vi "SoftwareGate_Rapid Read.vi"(0 "Timeout (s)":dbl, 1 "Channel":string="1", 2 "Digitizer Settings":T5={"Digitizer delay (us) "=0.0, "rf points per line"=2048, "lines per plane"=128, "Samp Rate (Hz)"=100000000.0, "Additional dig delay (us)"=0.0, "Voltage Scale"=0.4, "Pre-Looks"=0, "Offset delay (us)"=0.0, "bits A/D"=8, "Avg Num"=1, "DigTimeOut"=5.0, "Rel Dig Delay"=0.0, "Dig Ch"=0, "LeCroyCluster"={"LeCroy Channels"=[TRUE, FALSE, FALSE, FALSE], "LC read pt offset"=0.0, "Sweep Avg"=FALSE}, "Main Digitizer"=enum."NI Digitizer", "Dig Config"=enum."Single channel", "Digitizer ID Cluster"={"Acqiris/Alazar/SP ID"=[], "NI Instr Handles"=[], "LeCroy VISA"="", "GaGe Handle"={"Handle"=0, "Sample size"=0, "Resolution"=0, "Offset"=0, "Channels"=0, "Boards"=0}, "ATS Ref"="ATS9350", "Acqiris Address"=["PCI::INSTR0"], "ADQRef"=refnum, "adq_cu_ptr"=refnum}, "Trigger Settings"={"Trig Source"=1, "Trig Coupling"=0, "Trig Slope"=0, "Level (mV)"=1500.0}, "Bulk Acq"=FALSE, "Bulk Start Indexes"=[], "Data Ref RF"=refnum, "NI ID/Channel"=[], "Total Dig CH"=5, "Xtra Ann Trig delay (us)"=10.0, "Fix Z Delay?"=FALSE, "One Way Transmission?"=FALSE, "Data Ref Log"=refnum} {"Trigger Settings"."Trig Slope" items=["Positive", "Negative"]; "Trigger Settings"."Level (mV)" format="%.2f"; "Trigger Settings"."Trig Coupling" items=["DC 1 MOhm", "AC 1 MOhm", "DC 50 Ohm", "AC 50 Ohm"]; "Trigger Settings"."Trig Source" items=["Chan 1", "External"]; "Rel Dig Delay" format="%.2f"; "DigTimeOut" format="%.2f"; "Avg Num" min=1; "Offset delay (us)" format="%.2f"; "Additional dig delay (us)" format="%.2f"; "Digitizer delay (us)" format="%.2f"}, 7 "AlazarCluster":T9, 9 "Motion Settings":T1={"No Motion?"=FALSE, "Motion System"=enum."NI 735x", "Motion Bd ID"=1, "Motion Profile"="SMAC1", "# Axis"=1, "Reverse Z axis?"=TRUE, "SMAC Axis"=0, "scan pair"=enum."y-(x) scan", "RT fps"=6.0, "Steps per mm"=[1000, 1000, 1000, 1000], "Motor Parameters"={"velocity ct/s"=[10000.0, 10000.0, 10000.0, 50000.0], "accel ct/s^2"=[50000.0, 50000.0, 50000.0, 200000.0]}, "One Way Scan"=FALSE, "Reverse One Way Scan"=FALSE, "Global Position (mm)"=[], "Plane"=0, "Distance between\nscan lines (um)"=0.0, "Distance between\nscan planes (um)"=0.0, "number of scan planes"=1, "Total steps in line"=0, "Xtra plane\ndistance  (um)"=100, "Xtra planes "=1, "Add Axis"=FALSE, "overshoot cts"=200, "BKPT Shift"=0, "Scan Start Time (ms)"=0, "ESP VISA"="GPIB::1::INSTR", "3rd Axis"=1, "GL Ref Out"=refnum, "Galil Address"=""} {"3rd Axis" items=["x", "y", "z", "w"]; "Xtra planes" min=1; "Xtra plane\ndistance  (um)" min=0; "Distance between\nscan planes (um)" format="%.2f"; "Distance between\nscan lines (um)" format="%.2f"; "SMAC Axis" items=["None"=0, "Axis 1"=1, "Axis 2"=2, "Axis 3"=3, "Axis 4"=4, "Axis 5"=5, "Axis 6"=6, "Axis 7"=7, "Axis 8"=8, "Vector Space 1"=17, "Vector Space 2"=18, "Vector Space 3"=19, "Vector Space 4"=20]; "Motion Bd ID" min=1 max=32 step=1}, 11 "error in":errorcluster, 14 "Software Gate":bool) -> (3 "gain":dbl, 4 "Array":i16[][](array[numeric]), 6 "Reverse?":bool, 15 "error out":errorcluster)   [LabVIEW 2022 SP3]
uses:
  ScanningControl/Digitizers/-DigitizerRoutines/DigitizerSettings.ctl
  ScanningControl/Digitizers/-DigitizerRoutines/Digitizer.ctl
  ScanningControl/Digitizers/-DigitizerRoutines/DigConfig.ctl
  ScanningControl/Digitizers/-DigitizerRoutines/DigitizerID.ctl
  C:/Windows/System32/ADQAPI_dotNet_helper.dll
  ScanningControl/Motion Controllers/NI_controller/-NI_MotionRoutines/MotionParameters.ctl
  ScanningControl/Motion Controllers/NI_controller/-NI_MotionRoutines/MotionSys.ctl
  ScanningControl/Motion Controllers/-MotionRoutines/ScanAxis.ctl
  ScanningControl/Motion Controllers/-MotionRoutines/3rdAxis.ctl
  <vilib>/DAQmx/write.llb/DAQmx Write (Digital Bool 1Line 1Point).vi
  ScanningControl/Motion Controllers/-MotionRoutines/MotionGlobals.vi
  <vilib>/DAQmx/miscellaneous.llb/DAQmx Fill In Error Info.vi
  <instrlib>/niScope/Acquire/Fetch/niScope Multi Fetch Binary 8.vi
  <instrlib>/Acqiris Dx/Acqiris Dx.lvlib
panel:
  # "1-D and 2-D B scan settings"
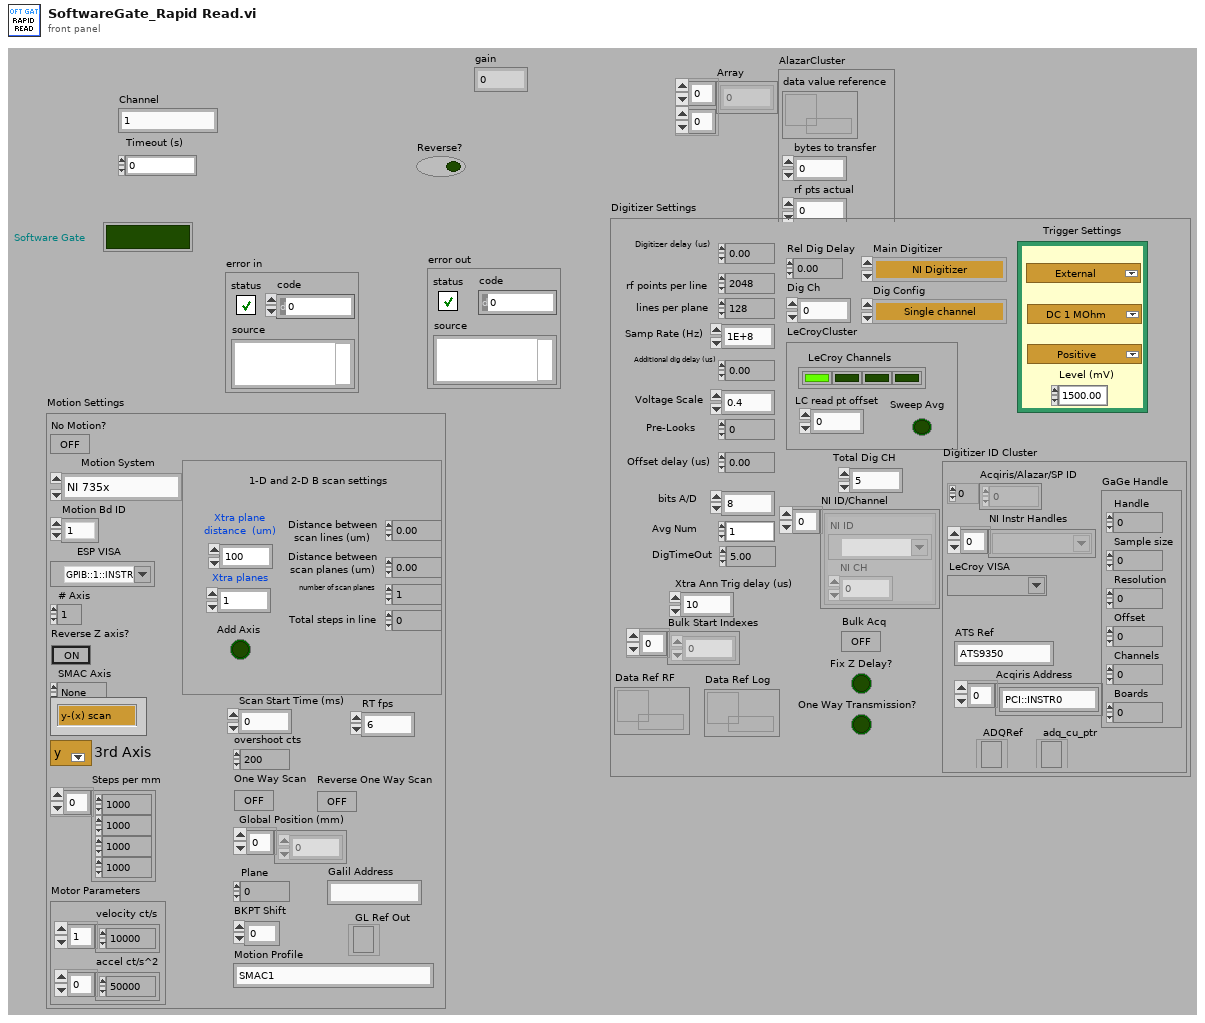
[diagram p1: front panel]
types:
  T1 = typedef "MotionParameters.ctl" = cluster{"No Motion?":bool, "Motion System":T2, "Motion Bd ID":u8, "Motion Profile":string, "# Axis":i8, "Reverse Z axis?":bool, "SMAC Axis":u16, "scan pair":T3, "RT fps":sgl, "Steps per mm":i32[], "Motor Parameters":cluster{"velocity ct/s":dbl[], "accel ct/s^2":dbl[]}, "One Way Scan":bool, "Reverse One Way Scan":bool, "Global Position (mm)":dbl[], "Plane":i32, "Distance between\nscan lines (um)":sgl, "Distance between\nscan planes (um)":sgl, "number of scan planes":i32, "Total steps in line":i32, "Xtra plane\ndistance  (um)":i32, "Xtra planes ":i32, "Add Axis":bool, "overshoot cts":i32, "BKPT Shift":i32, "Scan Start Time (ms)":u32, "ESP VISA":refnum<visa-resource-name>, "3rd Axis":T4, "GL Ref Out":refnum<k7>, "Galil Address":string}
  T2 = typedef "MotionSys.ctl" = enum16{"MM3000", "NI 735x", "Newport ESP", "No Motion Card", "Galil"}
  T3 = typedef "ScanAxis.ctl" = enum16{"y-(x) scan", "x-(y) scan", "z-(x) scan", "z-(y) scan", "y-(z) scan", "x-(z) scan", "w-(x) scan", "w-(y) scan", "w-(z) scan", "x-(w) scan", "y-(w) scan", "z-(w) scan"}
  T4 = typedef "3rdAxis.ctl" = u16
  T5 = typedef "DigitizerSettings.ctl" = cluster{"Digitizer delay (us) ":dbl, "rf points per line":i32, "lines per plane":i32, "Samp Rate (Hz)":dbl, "Additional dig delay (us)":dbl, "Voltage Scale":dbl, "Pre-Looks":i32, "Offset delay (us)":dbl, "bits A/D":i8, "Avg Num":i32, "DigTimeOut":sgl, "Rel Dig Delay":sgl, "Dig Ch":i32, "LeCroyCluster":cluster{"LeCroy Channels":bool[], "LC read pt offset":dbl, "Sweep Avg":bool}, "Main Digitizer":T6, "Dig Config":T7, "Digitizer ID Cluster":T8, "Trigger Settings":cluster{"Trig Source":u16, "Trig Coupling":u16, "Trig Slope":u16, "Level (mV)":dbl}, "Bulk Acq":bool, "Bulk Start Indexes":i32[], "Data Ref RF":refnum<data-value>, "NI ID/Channel":cluster{"NI ID":refnum<k15>, "NI CH":i32}[], "Total Dig CH":i32, "Xtra Ann Trig delay (us)":dbl, "Fix Z Delay?":bool, "One Way Transmission?":bool, "Data Ref Log":refnum<data-value>}
  T6 = typedef "Digitizer.ctl" = enum16{"Acqiris Digitizer", "NI Digitizer", "LeCroy", "GaGe", "AlazarTech", "No Digitizer", "Teledyne"}
  T7 = typedef "DigConfig.ctl" = enum16{"Single channel", "2 Chans w/ 2 Acqiris", "2 Chans w/ 1 Acqiris", "5-CH Pulser New", "5-CH pulser w/ ann array", "5-pass style ann array", "Empty"}
  T8 = typedef "DigitizerID.ctl" = cluster{"Acqiris/Alazar/SP ID":u32[], "NI Instr Handles":refnum<k15>[], "LeCroy VISA":refnum<visa-resource-name>, "GaGe Handle":cluster{"Handle":u32, "Sample size":u32, "Resolution":i32, "Offset":i32, "Channels":u32, "Boards":u32}, "ATS Ref":string, "Acqiris Address":string[], "ADQRef":refnum<k24>, "adq_cu_ptr":refnum<k24>}
  T9 = cluster{"data value reference":refnum<data-value>, "bytes to transfer":u32, "rf pts actual":u32}
  T10 = typedef "Var" = u8
  T11 = cluster{"horPos":dbl, "timeStampLo":u32, "timeStampHi":u32}[]
  T12 = cluster{"returnedSamplesPerSeg":i32, "indexFirstPoint":i32, "sampTime":dbl, "vGain":dbl, "vOffset":dbl, "returnedSegments":i32, "nbrAvgWforms":i32, "actualTriggersInAcqLo":u32, "actualTriggersInAcqHi":u32, "reserved3":dbl, "actualDataSize":u32, "missingValue":dbl}
  T13 = typedef "Bd Id Out" = u8
  T14 = cluster{"actualSamples":i32, "absoluteInitialX":dbl, "relativeInitialX":dbl, "xIncrement":dbl, "offset":dbl, "gain":dbl, "reserved1":dbl, "reserved2":dbl}[]
  T15 = cluster{"actualSamples":i32, "absoluteInitialX":dbl, "relativeInitialX":dbl, "xIncrement":dbl, "offset":dbl, "gain":dbl, "reserved1":dbl, "reserved2":dbl}
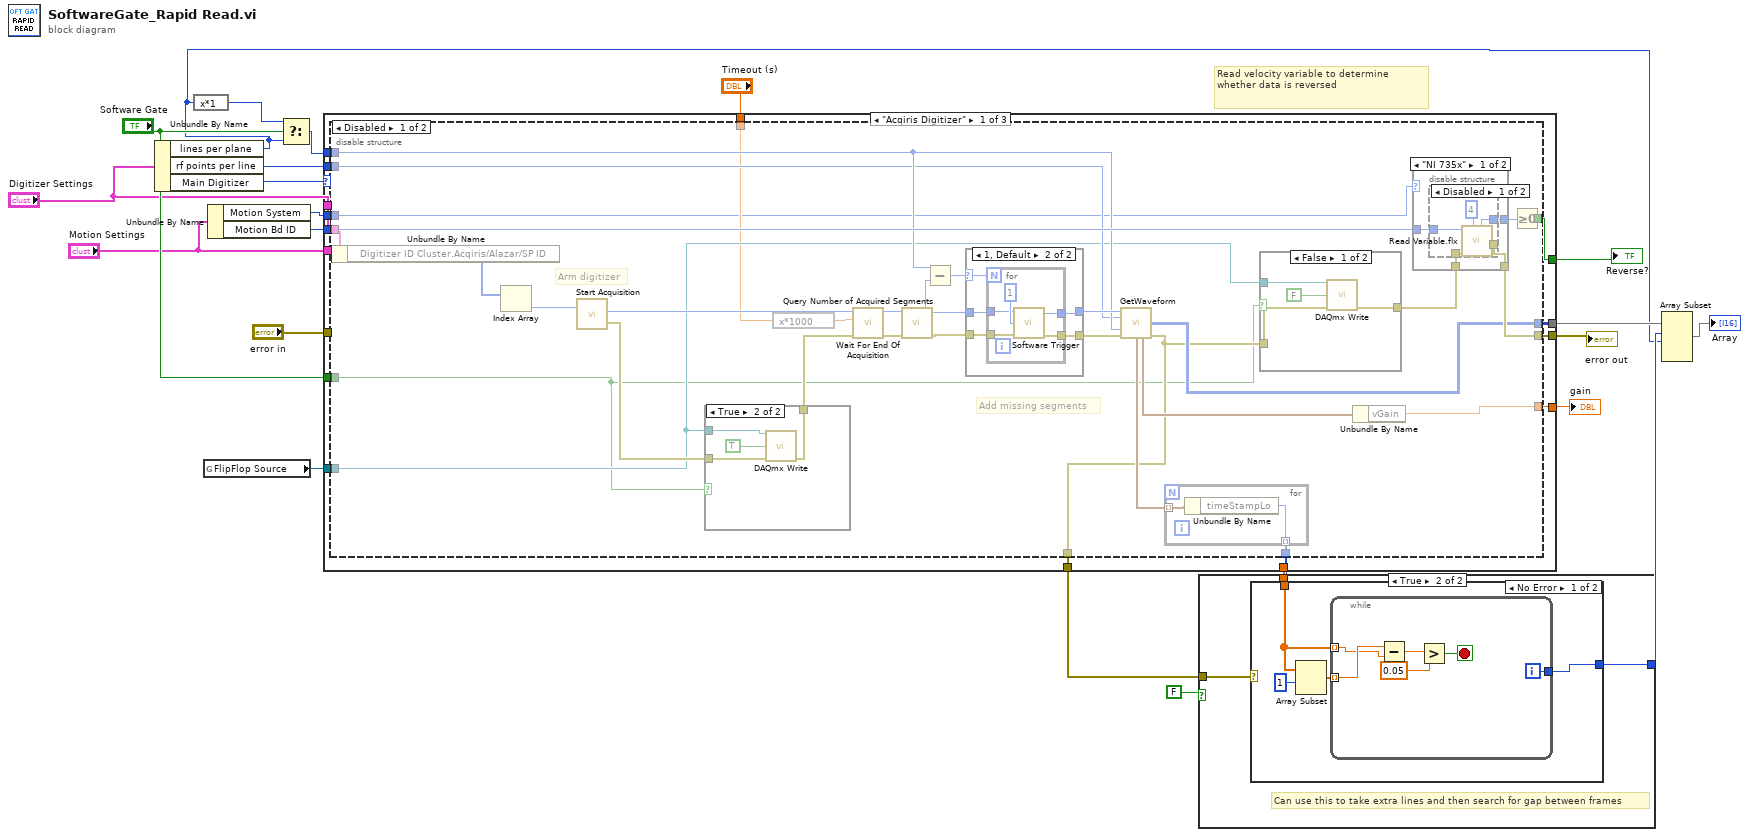
[diagram p0: block diagram]
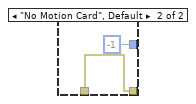
[diagram p7: hidden frame]
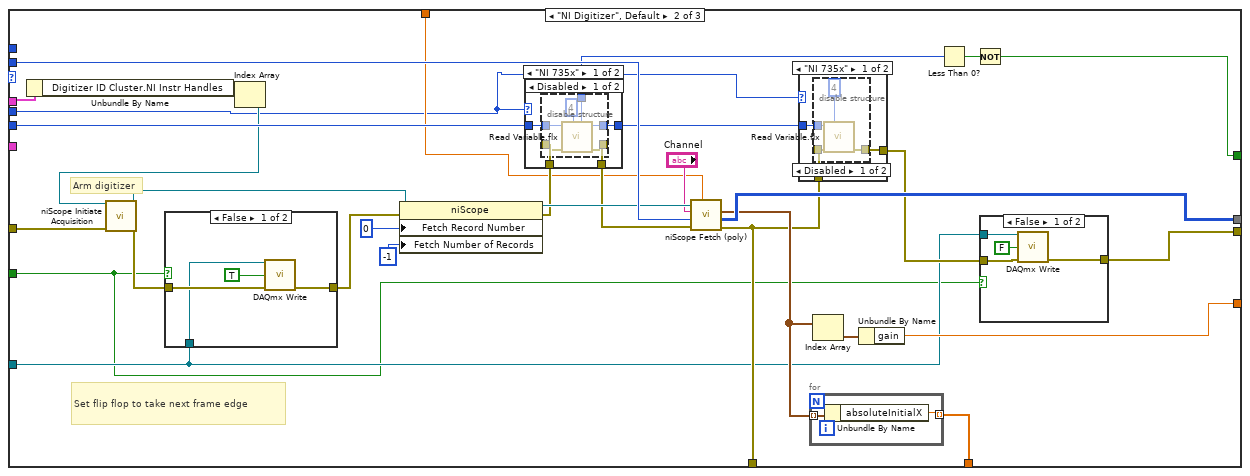
[diagram p10: hidden frame]
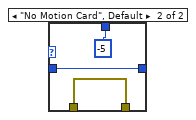
[diagram p16: hidden frame]
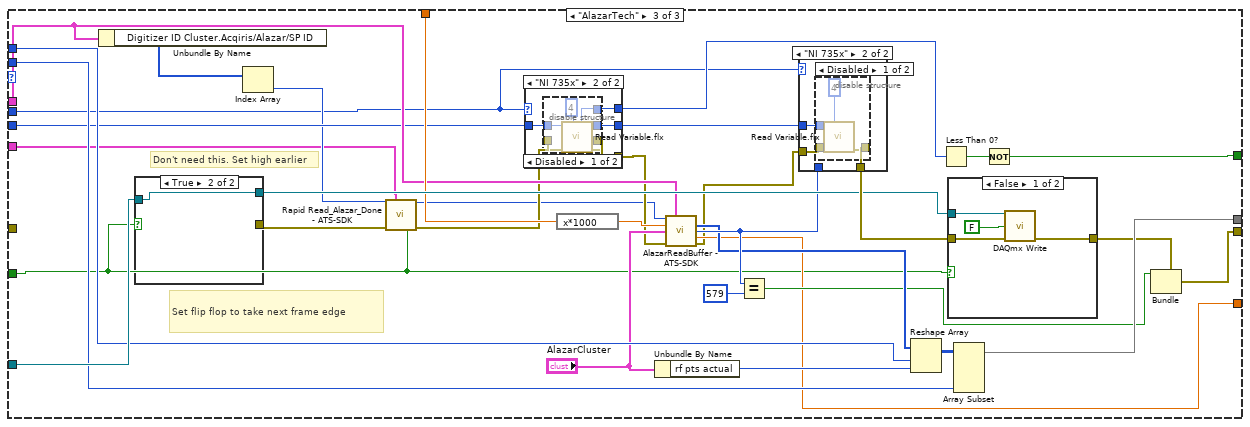
[diagram p17: hidden frame]
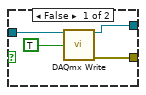
[diagram p18: hidden frame]
diagram:
  # "Read velocity variable to determine whether data is reversed"
  n1 = Unbundle By Name("Digitizer Settings") -> ("lines per plane"=w4:i32, "rf points per line"=w5:i32, "Main Digitizer"=w6:T6)
  n2 = expression code="x*1"(w4) -> (w16:i32)
  n3 = global read "MotionGlobals.vi" "FlipFlop Source"() -> (w18:refnum<k21>)
  n4 = Unbundle By Name("Motion Settings") -> ("Motion System"=w1:T2, "Motion Bd ID"=w2:u8)
  n5 = Select(t=w16, s="Software Gate", f=w4) -> (s? t:f=w15:i32)
  n6 = case shown="\"Acqiris Digitizer\"" w6 {
    tunnel: [w36 w107 w185] -> w22
    tunnel: w2 -> [w34 w133 w173]
    tunnel: "error in" -> [_ w131 _]
    tunnel: w5 -> [w32 w134 w194]
    tunnel: w15 -> [w33 _ w195]
    tunnel: [w31 w119 w193] -> w13
    tunnel: [w35 w116 w197] -> w20
    tunnel: [w30 w125 w182] -> w19
    tunnel: w18 -> [w29 w106 w200]
    tunnel: "Digitizer Settings" -> [w28 w115 w181]
    tunnel: "Timeout (s)" -> [w27 w110 w189]
    tunnel: [w26 w111 _] -> w14
    tunnel: [w25 w109 _] -> w10
    tunnel: "Software Gate" -> [w24 w105 w174]
    tunnel: "Motion Settings" -> [_ _ w170]
    tunnel: w1 -> [w23 w104 w169]
    frame "Acqiris Digitizer" {
      n7 = disable-structure shown="Disabled" {
        disable-tunnel: [w58 _] -> w36
        disable-tunnel: [w57 _] -> w35
        disable-tunnel: w34 -> [w56 _]
        disable-tunnel: w33 -> [w55 _]
        disable-tunnel: w32 -> [w54 _]
        disable-tunnel: [w53 _] -> w31
        disable-tunnel: [w51 _] -> w30
        disable-tunnel: w29 -> [w47 _]
        disable-tunnel: w28 -> [w46 _]
        disable-tunnel: w27 -> [w43 _]
        disable-tunnel: [w41 _] -> w26
        disable-tunnel: [w39 _] -> w25
        disable-tunnel: w24 -> [w38 _]
        disable-tunnel: w23 -> [w37 _]
        frame Disabled {
          # "Arm digitizer"
          # "Add missing segments"
          n8 = Unbundle By Name(w46) -> ("Digitizer ID Cluster.Acqiris/Alazar/SP ID"=w45:u32[])
          n9 = Index Array(array=w45) -> (element=w44:u32)  [unwired: 1 in]
          n10 = call <instrlib>:"Start Acquisition.vi"("Instrument ID"=w44) -> ("error out"=w50:errorcluster, "dup Instrument ID"=w60:u32)  [unwired: 3 in]
          n11 = case shown="True" w38 {
            tunnel: w50 -> [w74 w77]
            tunnel: [w74 w76] -> w49
            tunnel: w47 -> [_ w75]
            frame False {
            }
            frame True {
              n12 = call-poly <vilib>:"DAQmx Write.vi"("task/channels in"=w75, "data"=TRUE ("stop (T)"), "error in"=w77) -> ("error out"=w76:errorcluster)  [unwired: 10 in, 2 out]
            }
          }
          n13 = expression code="x*1000"(w43) -> (w40:dbl)
          n14 = call <instrlib>:"Wait For End Of Acquisition.vi"("error in (no error)"=w49, "Timeout"=w40, "Instrument ID"=w60) -> ("error out"=w61:errorcluster, "dup Instrument ID"=w65:u32)  [unwired: 3 out]
          n15 = call <instrlib>:"Query Number of Acquired Segments.vi"("error in (no error)"=w61, "Instrument ID"=w65) -> ("error out"=w67:errorcluster, "Number of Segments"=w68:i32, "dup Instrument ID"=w64:u32)  [unwired: 3 out]
          n16 = Subtract(x=w55, y=w68) -> (x-y=w63:i32)
          n17 = case shown="1, Default" w63 {
            selector: w63 -> [_ w94]
            tunnel: w67 -> [w92 w98]
            tunnel: [w92 w97] -> w66
            tunnel: w64 -> [w93 w96]
            tunnel: [w93 w95] -> w62
            frame 0 {
            }
            frame 1, Default {
              n18 = for {
                N: w94 -> [_]
                tunnel: w98 -> [w103]
                tunnel: w96 -> [w100]
                tunnel: [w102] -> w97
                tunnel: [w99] -> w95
                n19 = call <instrlib>:"Software Trigger.vi"("error in (no error)"=w103, "Type"=1, "Instrument ID"=w100) -> ("error out"=w102:errorcluster, "dup Instrument ID"=w99:u32)
              }
            }
          }
          n20 = call "GetWaveform.vi"("Acq ID Out"=w62, "Num Samps"=w54, "Num Segs"=w55, "error in"=w66) -> ("Acquired Waveform16 bit"=w53:i16[][], "segDescArray out"=w42:T11, "dataDesc"=w52:T12, "error out"=w39:errorcluster)  [unwired: 2 in, 6 out]
          n21 = for {
            tunnel: w42 -> [w80] mode=indexing
            tunnel: [w79] -> w41 mode=indexing
            n22 = Unbundle By Name(w80) -> ("timeStampLo"=w79:u32)
          }
          n23 = case shown="False" w38 {
            tunnel: [w71 w73] -> w48
            tunnel: w47 -> [w70 _]
            tunnel: w39 -> [w69 w73]
            frame False {
              n24 = call-poly <vilib>:"DAQmx Write.vi"("task/channels in"=w70, "data"=FALSE ("stop (T)"), "error in"=w69) -> ("error out"=w71:errorcluster)  [unwired: 10 in, 2 out]
            }
            frame True {
            }
          }
          n25 = Unbundle By Name(w52) -> ("vGain"=w51:dbl)
          n26 = case shown="\"NI 735x\"" w37 {
            tunnel: [w84 -1 ("Output")] -> w59
            tunnel: [w83 w91] -> w58
            tunnel: w56 -> [w82 _]
            tunnel: w48 -> [w81 w91]
            frame "NI 735x" {
              n27 = disable-structure shown="Disabled" {
                disable-tunnel: [w89 _] -> w84
                disable-tunnel: [w87 _] -> w83
                disable-tunnel: w82 -> [w86 _]
                disable-tunnel: w81 -> [w85 _]
                frame Disabled {
                  n28 = call <vilib>:"Read Variable.flx"("Var"=T10 4, "error in (no error)"=w85, "Board ID"=w86) -> ("error out"=w87:errorcluster, "Output"=w89:i32)  [unwired: 1 in, 4 out]
                }
                frame Enabled {
                }
              }
            }
            frame "No Motion Card", Default {
            }
          }
          n29 = Greater Or Equal To 0?(x=w59) -> (x >= 0?=w57:bool)
        }
        frame Enabled {
        }
      }
    }
    frame "NI Digitizer", Default {
      # "Set flip flop to take next frame edge"
      # "Arm digitizer"
      n30 = Unbundle By Name(w115) -> ("Digitizer ID Cluster.NI Instr Handles"=w114:refnum<k15>[])
      n31 = Index Array(array=w114) -> (element=w113:refnum<k15>)  [unwired: 1 in]
      n32 = call <instrlib>:"niScope Initiate Acquisition.vi"("instrument handle"=w113, "error in"=w131) -> ("instrument handle out"=w132:refnum<k15>, "error out"=w121:errorcluster)  [unwired: 1 in, 11 out]
      n33 = case shown="False" w105 {
        tunnel: w121 -> [w142 w144]
        tunnel: [w141 w144] -> w120
        tunnel: w106 -> [w140 _]
        frame False {
          n34 = call-poly <vilib>:"DAQmx Write.vi"("task/channels in"=w140, "data"=TRUE ("stop (T)"), "error in"=w142) -> ("error out"=w141:errorcluster)  [unwired: 10 in, 2 out]
        }
        frame True {
        }
      }
      n35 = property class="niScope"(reference=w132, error in=w120, "Fetch Record Number"=0, "Fetch Number of Records"=-1) -> (reference out=w128:refnum<k15>, error out=w124:errorcluster)
      n36 = case shown="\"NI 735x\"" w104 {
        tunnel: w133 -> [w159 w168]
        tunnel: w124 -> [w158 w167]
        tunnel: [w157 w167] -> w123
        tunnel: [w156 w168] -> w118
        tunnel: [w155 -5 ("Output")] -> w117
        frame "NI 735x" {
          n37 = disable-structure shown="Disabled" {
            disable-tunnel: w159 -> [w164 _]
            disable-tunnel: w158 -> [w163 _]
            disable-tunnel: [w162 _] -> w157
            disable-tunnel: [w161 _] -> w156
            disable-tunnel: [w160 _] -> w155
            frame Disabled {
              n38 = call <vilib>:"Read Variable.flx"("Var"=T10 4, "error in (no error)"=w163, "Board ID"=w164) -> ("error out"=w162:errorcluster, "Bd ID Out"=w161:T13, "Output"=w160:i32)  [unwired: 1 in, 3 out]
            }
            frame Enabled {
            }
          }
        }
        frame "No Motion Card", Default {
        }
      }
      n39 = call-poly <instrlib>:"niScope Fetch (poly).vi"("timeout"=w110, "error in"=w123, "numSamples"=w134, "channels"="Channel", "instrument handle"=w128) -> ("error out"=w109:errorcluster, "wfm"=w119:i8[][], "wfm info"=w112:T14)  [unwired: 4 out]
      n40 = case shown="\"NI 735x\"" w104 {
        tunnel: w109 -> [w149 w154]
        tunnel: [w148 w154] -> w108
        tunnel: w118 -> [w147 _]
        frame "NI 735x" {
          n41 = disable-structure shown="Disabled" {
            disable-tunnel: w149 -> [w152 _]
            disable-tunnel: [w151 _] -> w148
            disable-tunnel: w147 -> [w150 _]
            frame Disabled {
              n42 = call <vilib>:"Read Variable.flx"("Var"=T10 4, "error in (no error)"=w152, "Board ID"=w150) -> ("error out"=w151:errorcluster)  [unwired: 1 in, 5 out]
            }
            frame Enabled {
            }
          }
        }
        frame "No Motion Card", Default {
        }
      }
      n43 = for {
        tunnel: w112 -> [w146] mode=indexing
        tunnel: [w145] -> w111 mode=indexing
        n44 = Unbundle By Name(w146) -> ("absoluteInitialX"=w145:dbl)
      }
      n45 = Index Array(array=w112) -> (element=w127:T15)  [unwired: 1 in]
      n46 = Unbundle By Name(w127) -> ("gain"=w125:dbl)
      n47 = Less Than 0?(x=w117) -> (x < 0?=w122:bool)
      n48 = Not(x=w122) -> (.not. x?=w116:bool)
      n49 = case shown="False" w105 {
        tunnel: w108 -> [w137 w139]
        tunnel: [w136 w139] -> w107
        tunnel: w106 -> [w135 _]
        frame False {
          n50 = call-poly <vilib>:"DAQmx Write.vi"("task/channels in"=w135, "data"=FALSE ("stop (T)"), "error in"=w137) -> ("error out"=w136:errorcluster)  [unwired: 10 in, 2 out]
        }
        frame True {
        }
      }
    }
    frame "AlazarTech" {
      # "Don't need this. Set high earlier"
      # "Set flip flop to take next frame edge"
      n51 = Unbundle By Name(w181) -> ("Digitizer ID Cluster.Acqiris/Alazar/SP ID"=w190:u32[])
      n52 = case shown="True" w174 {
        tunnel: w200 -> [w205 w207]
        tunnel: [w204 _] -> w171
        tunnel: [w203 w207] -> w191
        frame False {
          n53 = call-poly <vilib>:"DAQmx Write.vi"("task/channels in"=w205, "data"=TRUE ("stop (T)")) -> ("task out"=w203:refnum<k21>, "error out"=w204:errorcluster)  [unwired: 11 in, 1 out]
        }
        frame True {
        }
      }
      n54 = Index Array(array=w190) -> (element=w172:u32)  [unwired: 1 in]
      n55 = call "Rapid Read_Alazar_Done - ATS-SDK.vi"("Handle"=w172, "Motion Settings"=w170, "error out"=w171, "Pause?"=w174) -> ("Handle Out"=w175:u32, "error out"=w176:errorcluster)  [unwired: 9 in, 1 out]
      n56 = case shown="\"NI 735x\"" w169 {
        tunnel: w173 -> [w223 w228]
        tunnel: w176 -> [w221 w227]
        tunnel: [w223 w226] -> w199
        tunnel: [-5 ("Output") w225] -> w198
        tunnel: [w221 w224] -> w178
        frame "No Motion Card", Default {
        }
        frame "NI 735x" {
          n57 = disable-structure shown="Disabled" {
            disable-tunnel: w228 -> [w233 _]
            disable-tunnel: w227 -> [w232 _]
            disable-tunnel: [w231 _] -> w226
            disable-tunnel: [w230 _] -> w225
            disable-tunnel: [w229 _] -> w224
            frame Disabled {
              n58 = call <vilib>:"Read Variable.flx"("Var"=T10 4, "error in (no error)"=w232, "Board ID"=w233) -> ("error out"=w229:errorcluster, "Bd ID Out"=w231:T13, "Output"=w230:i32)  [unwired: 1 in, 3 out]
            }
            frame Enabled {
            }
          }
        }
      }
      n59 = expression code="x*1000"(w189) -> (w180:dbl)
      n60 = Unbundle By Name("AlazarCluster") -> ("rf pts actual"=w196:u32)
      n61 = call "AlazarReadBuffer - ATS-SDK.vi"("Handle"=w175, "Digitizer Settings"=w181, "time out (ms)"=w180, "AlazarCluster"="AlazarCluster", "error in (no error)"=w178) -> ("Data Array"=w184:i16[], "Return Code"=w187:u32, "Voltage Scale"=w182:dbl, "error out"=w177:errorcluster)  [unwired: 6 in, 1 out]
      n62 = Equal?(x=w187, y=u32 579) -> (x = y?=w183:bool)
      n63 = case shown="\"NI 735x\"" w169 {
        tunnel: w187 -> [_ _]
        tunnel: [w213 w216] -> w201
        tunnel: w199 -> [_ w215]
        tunnel: w177 -> [w213 w214]
        frame "No Motion Card", Default {
        }
        frame "NI 735x" {
          n64 = disable-structure shown="Disabled" {
            disable-tunnel: [w219 _] -> w216
            disable-tunnel: w215 -> [w218 _]
            disable-tunnel: w214 -> [w217 _]
            frame Disabled {
              n65 = call <vilib>:"Read Variable.flx"("Var"=T10 4, "error in (no error)"=w217, "Board ID"=w218) -> ("error out"=w219:errorcluster)  [unwired: 1 in, 5 out]
            }
            frame Enabled {
            }
          }
        }
      }
      n66 = Reshape Array(w184, w195, w196) -> (w192:i16[][])
      n67 = Less Than 0?(x=w198) -> (x < 0?=w202:bool)
      n68 = case shown="False" w174 {
        tunnel: w201 -> [w211 w212]
        tunnel: [w210 w212] -> w186
        tunnel: w191 -> [w208 _]
        frame False {
          n69 = call-poly <vilib>:"DAQmx Write.vi"("task/channels in"=w208, "data"=FALSE ("stop (T)"), "error in"=w211) -> ("error out"=w210:errorcluster)  [unwired: 10 in, 2 out]
        }
        frame True {
        }
      }
      n70 = Array Subset(array=w192, length (col)=w194) -> (w193:i16[][])  [unwired: 3 in]
      n71 = Not(x=w202) -> (.not. x?=w197:bool)
      n72 = Bundle(cluster=w186, "status"=w183) -> (w185:errorcluster)  [unwired: 2 in]
    }
  }
  "Reverse?" <- w20
  "error out" <- w22
  "gain" <- w19
  n73 = case shown="True" FALSE {
    tunnel: w14 -> [_ w237]
    tunnel: [_ w236] -> w12
    tunnel: w10 -> [_ w235]
    frame False {
    }
    frame True {
      # "Can use this to take extra lines and then search for gap between frames"
      n74 = case shown="No Error" w235 {
        tunnel: w237 -> [w241 _]
        tunnel: [w238 _] -> w236
        frame No Error {
          n75 = Array Subset(array=w241, index=1) -> (w239:dbl[])  [unwired: 1 in]
          n76 = while {
            tunnel: w241 -> [w246] mode=indexing
            tunnel: w239 -> [w247] mode=indexing
            tunnel: [w242] -> w238
            i -> [w242]
            stop <- w243 stop-if-true
            n77 = Subtract(x=w247, y=w246) -> (x-y=w245:dbl)
            n78 = Greater?(x=w245, y=0.05) -> (0:w243:bool)
          }
        }
        frame Error {
        }
      }
    }
  }
  n79 = Array Subset(array=w13, index (row)=w12, length (row)=w4) -> (→"Array":i16[][])  [unwired: 2 in]
